vi "TWM Client Cmd Get Versions.vi"(5 "timeout [ms] (3000)":i32=3000, 7 "end of packet key":string="TWM:command:EndOfPacket", 8 "error in":errorcluster, 11 "handle":i32) -> (0 "error out":errorcluster, 2 "TWM client version string":string, 3 "handle out":i32)   [LabVIEW 2020, in "TWM Client.lvlib"]
doc: "Retrieves version of TWM client and TWM itself."
uses:
  octave/infolib/GetString.vi
  <vilib>/ErrorRing/Error Ring.xnode
  TWM Client.lvlib
  octave/infolib/infolib.lvlib
  <vilib>/Utility/error.llb/Error Cluster From Error Code.vi
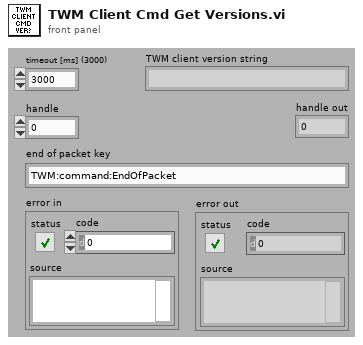
[diagram p1: front panel]
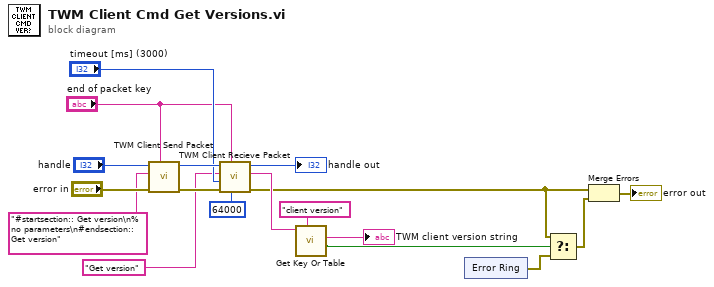
[diagram p0: block diagram]
diagram:
  n1 = call "TWM Client Send Packet.vi"("end of packet key"="end of packet key", "error in"="error in", "command string"="#startsection:: Get version\n% no parameters\n#endsection:: Get version", "handle"="handle") -> ("error out"=w13:errorcluster, "handle out"=w11:i32)  [unwired: 6 in]
  n2 = call "TWM Client Recieve Packet.vi"("max message length (1024)"=64000, "end of packet key"="end of packet key", "error in"=w13, "timeout [ms] (5000 ms)"="timeout [ms] (3000)", "message header (empty)"="Get version" ("key string"), "handle in"=w11) -> ("error out"=w4:errorcluster, "message data"=w6:string, "handle out"=→"handle out":i32)  [unwired: 3 in]
  n3 = call-poly "Get Key Or Table.vi"("key description"="client version", "info data"=w6) -> ("key found?"=w1:bool, "value"=→"TWM client version string":string)  [unwired: 6 in, 2 out]
  n4 = xnode "Error Ring"() -> ("error out"=w5:errorcluster)
  n5 = Select(t=w4, s=w1, f=w5) -> (s? t:f=w3:errorcluster)
  n6 = Merge Errors(w4, w3) -> (→"error out":errorcluster)
